vi "LJM_NamesToAddresses.vi"(7 "NumFrames":i32, 8 "error in":errorcluster, 11 "aNames":string[](array[string])) -> (0 "error out":errorcluster, 2 "aTypes":i32[](array[numeric]), 3 "aAddresses":i32[](array[numeric]))   [LabVIEW 2017]
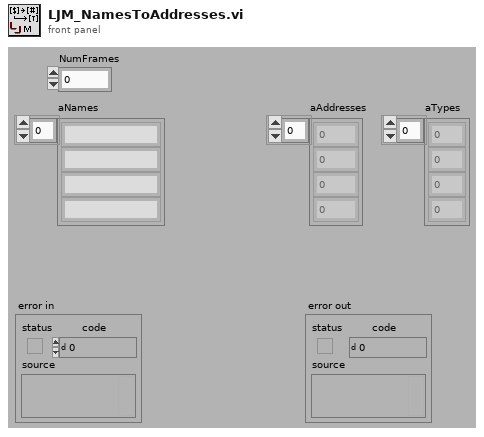
[diagram p1: front panel]
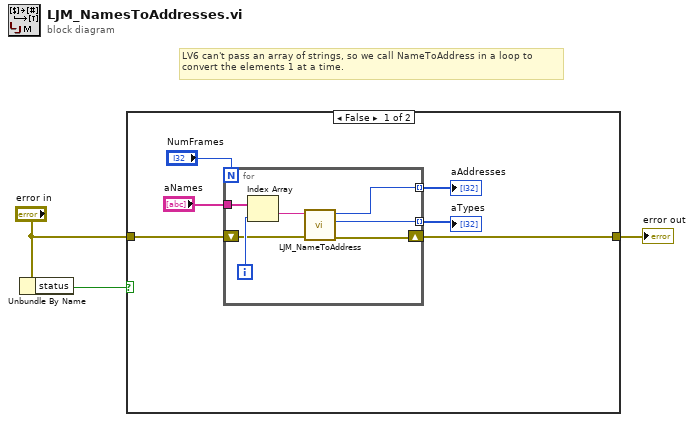
[diagram p0: block diagram]
diagram:
  # "LV6 can't pass an array of strings, so we call NameToAddress in a loop to\nconvert the elements 1 at a time."
  n1 = Unbundle By Name("error in") -> ("status"=w3:bool)
  n2 = case shown="False" w3 {
    tunnel: "error in" -> [w8 w17]
    tunnel: [w4 w17] -> w1
    frame False {
      n3 = for {
        N: "NumFrames" -> [_]
        tunnel: "aNames" -> [w15]
        shift-right: [w13] -> w4
        shift-left: w8 -> [w14]
        tunnel: [w11] -> w6 mode=indexing
        tunnel: [w10] -> w5 mode=indexing
        i -> [w16]
        n4 = Index Array(array=w15, index=w16) -> (element=w12:string)
        n5 = call "LJM_NameToAddress.vi"("error in"=w14, "Name"=w12) -> ("error out"=w13:errorcluster, "Type"=w11:i32, "Address"=w10:i32)  [unwired: 7 in]
      }
      "aAddresses" <- w5
      "aTypes" <- w6
    }
    frame True {
    }
  }
  "error out" <- w1
